vi "Set SPAN Component EPA.vi"(10 "EPA Optionsfeld":refnum<vi>, 11 "EPA Optionsfeld":T1) -> ()   [LabVIEW 2020, in "Linearisierung v2.lvlib" / "SpanEinstellungen.lvlib"]
uses:
  SpanEinstellungen.lvlib
  EPA Optionsfeld.ctl
  Linearisierung v2.lvlib
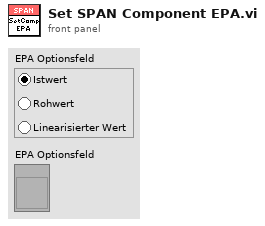
[diagram p1: front panel]
types:
  T1 = typedef "Linearisierung v2.lvlib/EPA Optionsfeld.ctl" = enum32{"Istwert", "Rohwert", "Linearisierter Wert"}
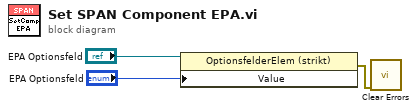
[diagram p0: block diagram]
diagram:
  n1 = property class="OptionsfelderElem (strikt)"(reference="EPA Optionsfeld", "Value"="EPA Optionsfeld") -> (error out=w3:errorcluster)  [unwired: 1 in, 1 out]
  n2 = call <vilib>:"Clear Errors.vi"("error in (no error)"=w3) -> ()  [unwired: 5 in, 2 out]
